vi "Example Basic.vi"() -> ()   [LabVIEW 2019]
doc: "Example to import or export JSON to LabVIEW Variants.\nCreated by: Ryan Pacini"
uses:
  lib/labview_json.lvlib
panel:
  out "Same?":bool
  out "Root":T1
  out "JSON":string
  in  "Root":T1={"squadName"="Super hero squad", "homeTown"="Metro City", "formed"=2016, "secretBase"="Super tower", "active"=TRUE, "members"=[{"name"="Molecule Man", "age"=29, "secretIdentity"="Dan Jukes", "powers"=["Radiation resistance", "Turning tiny", "Radiation blast"]}, {"name"="Madame Uppercut", "age"=39, "secretIdentity"="Jane Wilson", "powers"=["Million tonne punch", "Damage resistance", "Superhuman reflexes"]}, {"name"="Eternal Flame", "age"=1000000, "secretIdentity"="Unknown", "powers"=["Immortality", "Heat Immunity", "Inferno", "Teleportation", "Interdimensional travel"]}]}
  out "error out":errorcluster
  # "1. Variant to JSON"
  # "2. JSON to Variant"
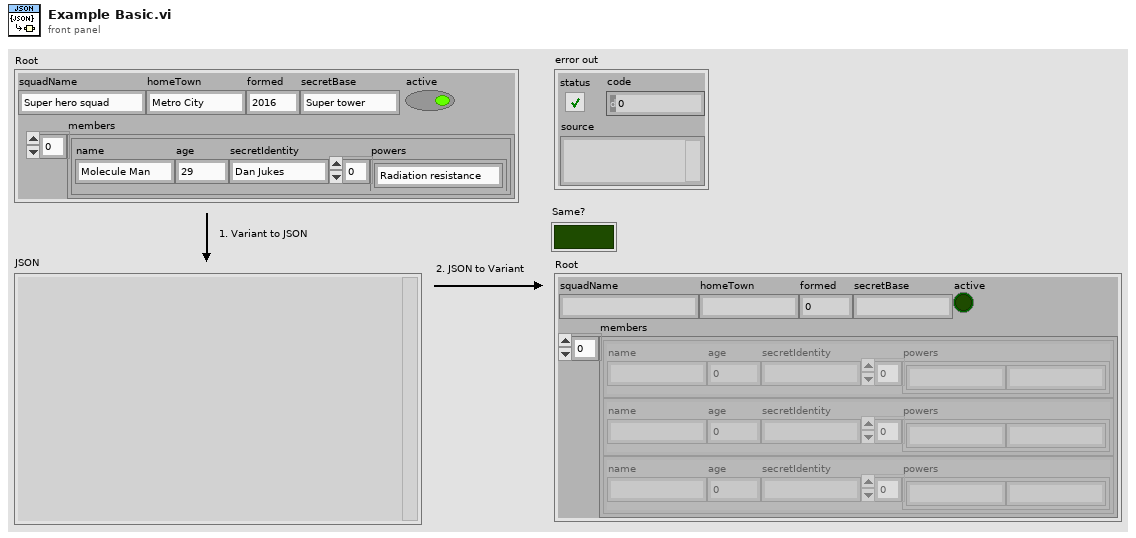
[diagram p1: front panel]
types:
  T1 = cluster{"squadName":string, "homeTown":string, "formed":i32, "secretBase":string, "active":bool, "members":cluster{"name":string, "age":i32, "secretIdentity":string, "powers":string[]}[]}
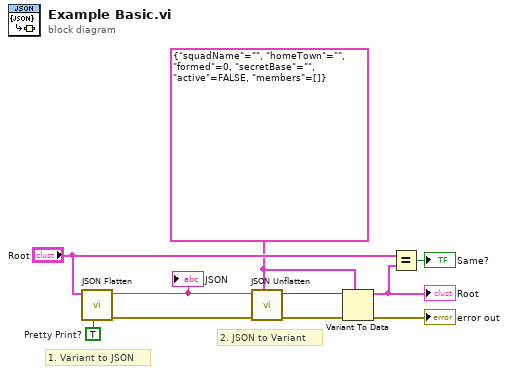
[diagram p0: block diagram]
diagram:
  w1 = T1 {"squadName"="", "homeTown"="", "formed"=0, "secretBase"="", "active"=FALSE, "members"=[]} ("Root")
  w2 = TRUE  # Pretty Print?
  # "2. JSON to Variant"
  # "1. Variant to JSON"
  n1 = call "JSON Flatten.vi"("Pretty Print? (F)"=w2, "Variant in"="Root") -> ("error out"=w8:errorcluster, "JSON out"=w10:string)  [unwired: 8 in]
  "JSON" <- w10
  n2 = call "JSON Unflatten.vi"("Variant Type"=w1, "error in (no error)"=w8, "JSON in"=w10) -> ("error out"=w9:errorcluster, "Variant out"=w6:variant)  [unwired: 6 in, 1 out]
  n3 = Variant To Data(error in=w9, type=w1, Variant=w6) -> (data=w5:T1, error out=→"error out":errorcluster)
  "Root" <- w5
  n4 = Equal?(x="Root", y=w5) -> (x = y?=→"Same?":bool)
